vi "Initi_stimuli.vi"(7 "XML Elements":string, 8 "error in (no error)":errorcluster, 9 "LstBox Refnum in":refnum<vi>, 10 "Clust Refnum":refnum<vi>, 11 "ListBox in":refnum<vi>) -> (0 "error IO":errorcluster, 3 "Array":T1(array[cluster]))   [LabVIEW 2016]
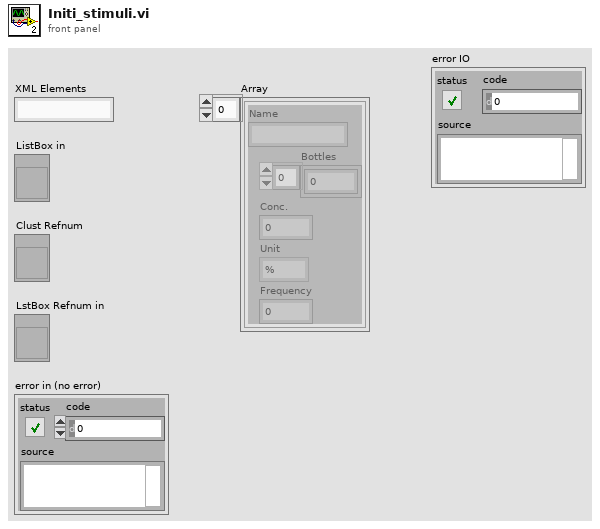
[diagram p1: front panel]
types:
  T1 = cluster{"Name":string, "Bottles":i32[], "Conc.":dbl, "Unit":enum16{"%", "ppm"}, "Frequency":dbl}[]
  T2 = cluster{"Name":string, "Bottles":i32[], "Conc.":dbl, "Unit":enum16{"%", "ppm"}, "Duration":dbl}[]
  T3 = cluster{"Name":string, "Bottles ":i32, "Conc.":dbl, "Unit":enum16{"%", "ppm"}, "Duration":dbl, "Add stimulus button":bool, "Remove stimulus button ":bool}
  T4 = cluster{"Name":string, "Bottles":i32[], "Conc.":dbl, "Unit":enum16{"%", "ppm"}, "Duration":dbl}
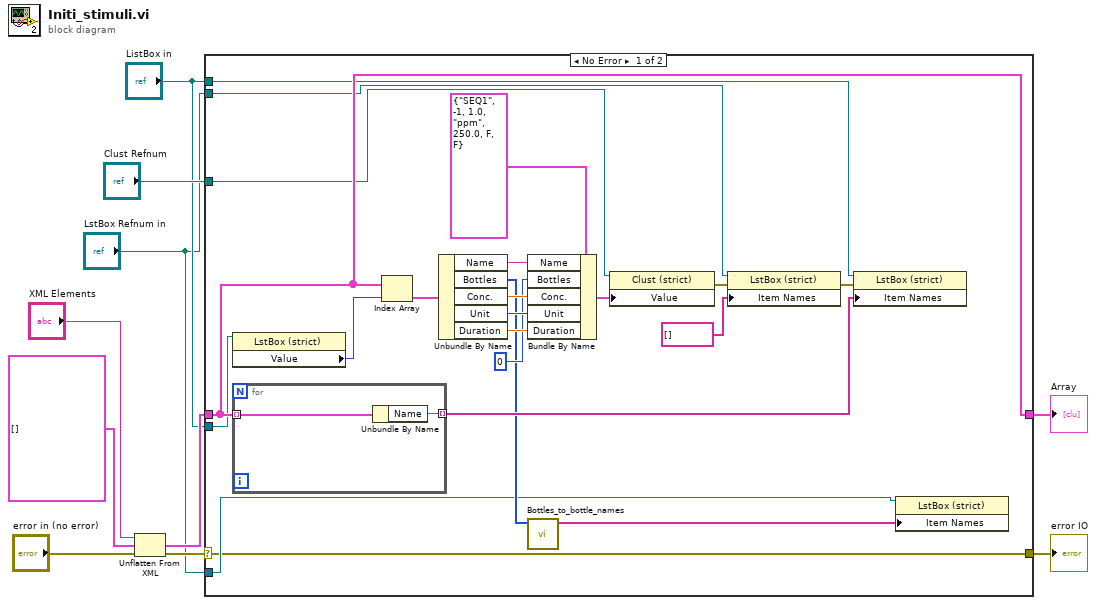
[diagram p0: block diagram]
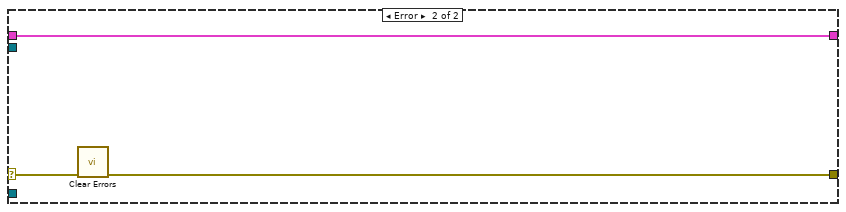
[diagram p2: hidden frame]
diagram:
  n1 = Unflatten From XML(xml string="XML Elements", type=T2 [], error in (no error)="error in (no error)") -> (value=w5:T2, error out=w6:errorcluster)
  n2 = case shown="No Error" w6 {
    selector: w6 -> [w11 w36]
    tunnel: [w28 w37] -> w10
    tunnel: w5 -> [w28 w37]
    tunnel: "ListBox in" -> [w16 _]
    tunnel: "Clust Refnum" -> [w15 _]
    tunnel: "LstBox Refnum in" -> [w14 _]
    tunnel: "ListBox in" -> [w13 _]
    tunnel: "LstBox Refnum in" -> [w12 _]
    tunnel: [w11 w35] -> w1
    frame No Error {
      n3 = property on="Property Node" class="LstBox (strict)"(reference=w13) -> ("Value"=w27:i32)  [unwired: 1 in, 2 out]
      n4 = for {
        tunnel: w28 -> [w34] mode=indexing
        tunnel: [w33] -> w32 mode=indexing
        n5 = Unbundle By Name(w34) -> ("Name"=w33:string)
      }
      n6 = Index Array(array=w28, index=w27) -> (element=w26:T4)
      n7 = Unbundle By Name(w26) -> ("Name"=w24:string, "Bottles"=w18:i32[], "Conc."=w23:dbl, "Unit"=w22:enum16{"%", "ppm"}, "Duration"=w21:dbl)
      n8 = Bundle By Name(cluster=T3 {"Name"="SEQ1", "Bottles "=-1, "Conc."=1.0, "Unit"=enum."ppm", "Duration"=250.0, "Add stimulus button"=FALSE, "Remove stimulus button "=FALSE} ("Stimulus properties"), "Name"=w24, "Bottles"=0, "Conc."=w23, "Unit"=w22, "Duration"=w21) -> (w20:T3)
      n9 = call "Bottles_to_bottle_names.vi"("Bottles"=w18) -> ("Array"=w17:string[])  [unwired: 10 in]
      n10 = property on="Property Node" class="Clust (strict)"(reference=w15, "Value"=w20) -> (error out=w30:errorcluster)  [unwired: 1 in, 1 out]
      n11 = property on="Property Node" class="LstBox (strict)"(reference=w14, error in=w30, "Item Names"=string[] []) -> (error out=w29:errorcluster)  [unwired: 1 out]
      n12 = property on="Property Node" class="LstBox (strict)"(reference=w16, error in=w29, "Item Names"=w32) -> ()  [unwired: 2 out]
      n13 = property on="Property Node" class="LstBox (strict)"(reference=w12, "Item Names"=w17) -> ()  [unwired: 1 in, 2 out]
    }
    frame Error {
      n14 = call <vilib>:"Clear Errors.vi"("error in (no error)"=w36) -> ("error out"=w35:errorcluster)  [unwired: 5 in, 1 out]
    }
  }
  "Array" <- w10
  "error IO" <- w1
